vi "Platform System Light.vi"(8 "error in (no error)":errorcluster, 10 "Enable Light State (F:Disabled)":bool, 11 "VISA resource name":refnum<visa-resource-name>) -> (0 "error out":errorcluster, 3 "VISA resource name out":refnum<visa-resource-name>)   [LabVIEW 2018, in "LTB-1.lvlib" / "3150.lvlib"]
doc: "Enables or disables the light of the device. When STATe OFF is selected, no device light is ON except source active LEDs."
uses:
  3150.lvlib
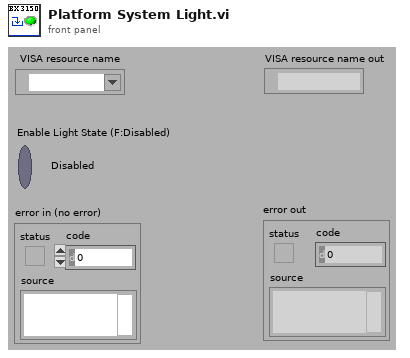
[diagram p1: front panel]
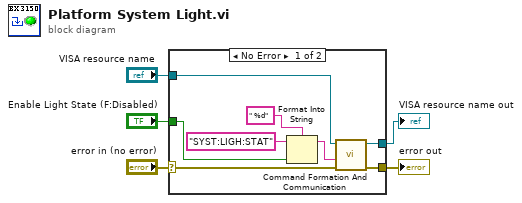
[diagram p0: block diagram]
diagram:
  n1 = case shown="No Error" "error in (no error)" {
    selector: "error in (no error)" -> [w12 w14]
    tunnel: "VISA resource name" -> [w13 w15]
    tunnel: [w11 w15] -> w4
    tunnel: [w10 w14] -> w3
    tunnel: "Enable Light State (F:Disabled)" -> [w8 _]
    frame No Error {
      n2 = Format Into String(format string=" %d", initial string="SYST:LIGH:STAT" ("Command"), w8) -> (resulting string=w6:string)  [unwired: 1 in, 1 out]
      n3 = call "Command Formation And Communication.vi"("error in (no error)"=w12, "Command"=w6, "VISA resource name"=w13) -> ("error out"=w10:errorcluster, "VISA resource name out"=w11:refnum<visa-resource-name>)  [unwired: 1 in, 6 out]
    }
    frame Error {
    }
  }
  "VISA resource name out" <- w4
  "error out" <- w3
